vi "V-Meter Measure (2182A).vi"(8 "error in (no error)":errorcluster, 11 "VISA resource name in":refnum<visa-resource-name>) -> (0 "error out":errorcluster, 2 "Measurement":dbl, 3 "VISA resource name out":refnum<visa-resource-name>)   [LabVIEW 2016, in "Hall Effect Library.lvlib"]
uses:
  Hall Effect Library.lvlib
  Global Variables/Test Settings.vi
  <instrlib>/Keithley 2182A/Keithley 2182A.lvlib
panel:
  out "Array":dbl[](array[numeric])
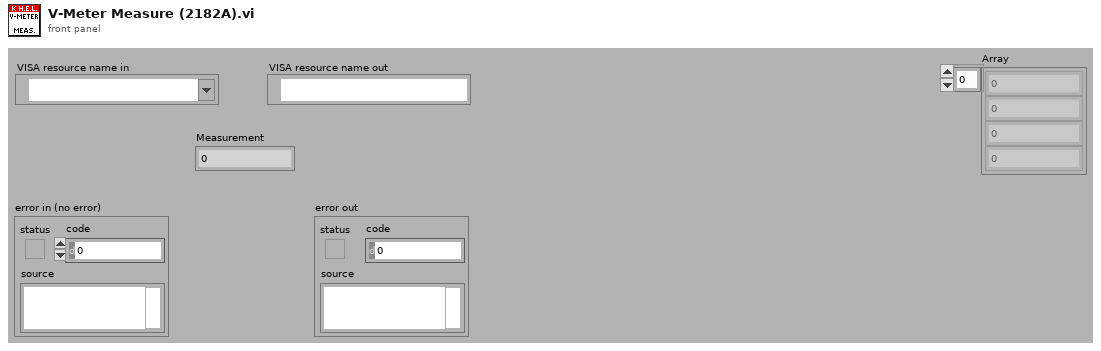
[diagram p1: front panel]
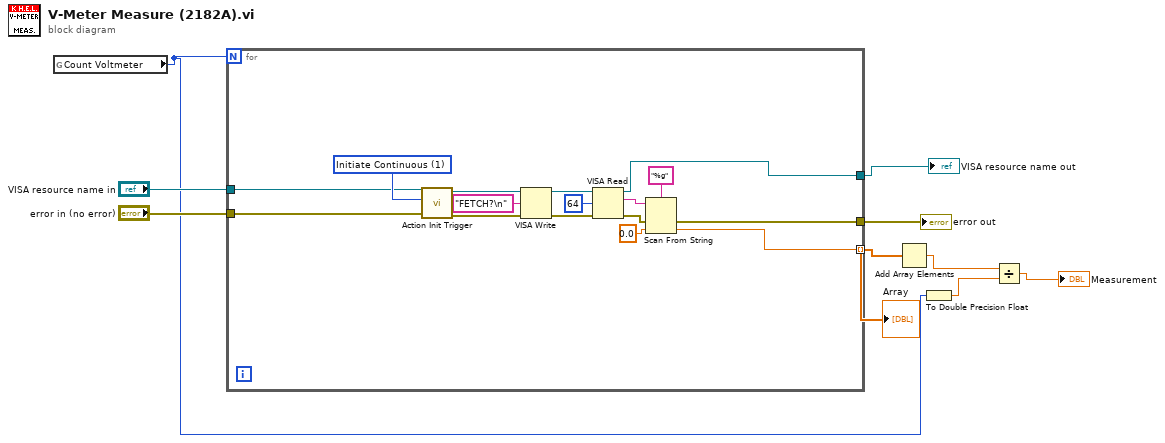
[diagram p0: block diagram]
diagram:
  n1 = global read "Test Settings.vi" "Count Voltmeter"() -> (w4:i32)
  n2 = for {
    N: w4 -> [_]
    tunnel: "VISA resource name in" -> [w14]
    tunnel: "error in (no error)" -> [w13]
    tunnel: [w12] -> w5 mode=indexing
    tunnel: [w11] -> w7
    tunnel: [w10] -> w6
    w25 = i16 1 items=["Don't Initiate"=-1, "Initiate Single"=0, "Initiate Continuous"=1] ("Inititiate Mode (Init Continuous)")
    n3 = call <instrlib>:"Action Init Trigger.vi"("error in"=w13, "Inititiate Mode (Init Continuous)"=w25, "VISA resource name"=w14) -> ("error out"=w17:errorcluster, "VISA resource name out"=w16:refnum<visa-resource-name>)  [unwired: 7 out]
    n4 = VISA Write(VISA resource name=w16, write buffer="FETCH?\n", error in (no error)=w17) -> (VISA resource name out=w19:refnum<visa-resource-name>, error out=w20:errorcluster)  [unwired: 1 out]
    n5 = VISA Read(VISA resource name=w19, byte count=u32 64, error in (no error)=w20) -> (VISA resource name out=w11:refnum<visa-resource-name>, read buffer=w22:string, error out=w15:errorcluster)  [unwired: 1 out]
    n6 = Scan From String(format string="%g", input string=w22, error in=w15, default 1=0.0 ("default value 1")) -> (error out=w10:errorcluster, output 1=w12:dbl)  [unwired: 1 in, 2 out]
  }
  "error out" <- w6
  "VISA resource name out" <- w7
  "Array" <- w5
  n7 = Add Array Elements(numeric array=w5) -> (sum=w3:dbl)
  n8 = To Double Precision Float(number=w4) -> (double precision float=w2:dbl)
  n9 = Divide(x=w3, y=w2) -> (x/y=→"Measurement":dbl)
